vi "Done.vi"(11 "State in":cluster{"Hallway":string[], "Rooms":string[][]}) -> (2 "Done?":bool, 3 "State out":cluster{"Hallway":string[], "Rooms":string[][]})   [LabVIEW 2019, in "23.lvlib"]
uses:
  23.lvlib
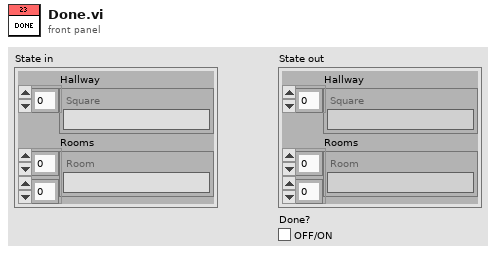
[diagram p1: front panel]
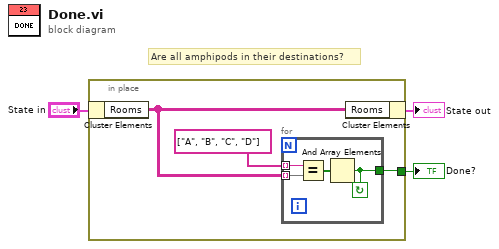
[diagram p0: block diagram]
diagram:
  # "Are all amphipods in their destinations?"
  n1 = in-place {
    in-place-border: [w4] -> w1
    n2 = in-place-cluster #1("State in") -> ("Rooms"=w6:string[][])
    n3 = for {
      tunnel: w6 -> [w8] mode=indexing
      tunnel: [w9] -> w4
      tunnel: string[] ["A", "B", "C", "D"] -> [w7] mode=indexing
      stop <- w9 continue-if-true
      n4 = Equal?(x=w7, y=w8) -> (x = y?=w10:bool[])
      n5 = And Array Elements(Boolean array=w10) -> (logical AND=w9:bool)
    }
    n6 = in-place-cluster #1("Rooms"=w6) -> (→"State out":cluster{"Hallway":string[], "Rooms":string[][]})
  }
  "Done?" <- w1
